vi "Get Channels Timing.vi"(8 "error in (no error)":errorcluster, 10 "group name in":string, 11 "Data file":T2) -> (0 "error out":errorcluster, 2 "Channels info":T1[](array[typedef]), 4 "Latest finish":dbl, 5 "Plots exist":bool, 6 "Earliest start":dbl)   [LabVIEW 2015]
uses:
  Controls/Channel name entry.ctl
  Controls/Data Viewer Entry.ctl
  Controls/TDMS channel info.ctl
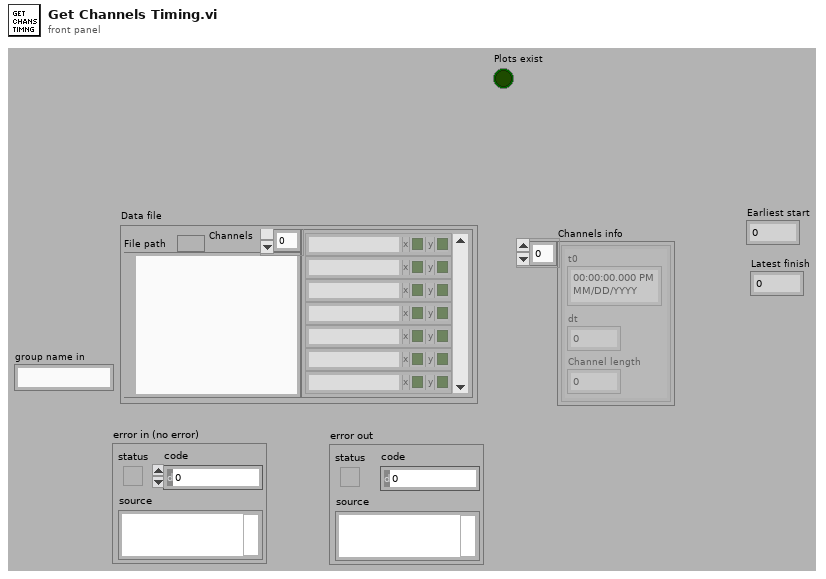
[diagram p1: front panel]
types:
  T1 = typedef "TDMS channel info.ctl" = cluster{"t0":timestamp, "dt":dbl, "Channel length":i64}
  T2 = typedef "Data Viewer Entry.ctl" = cluster{"File path":path, "Channels":T3[]}
  T3 = typedef "Channel name entry.ctl" = cluster{"Name":string, "x":bool, "y":bool}
  T4 = enum16{"open", "open or create", "create or replace", "create", "open (read-only)"}
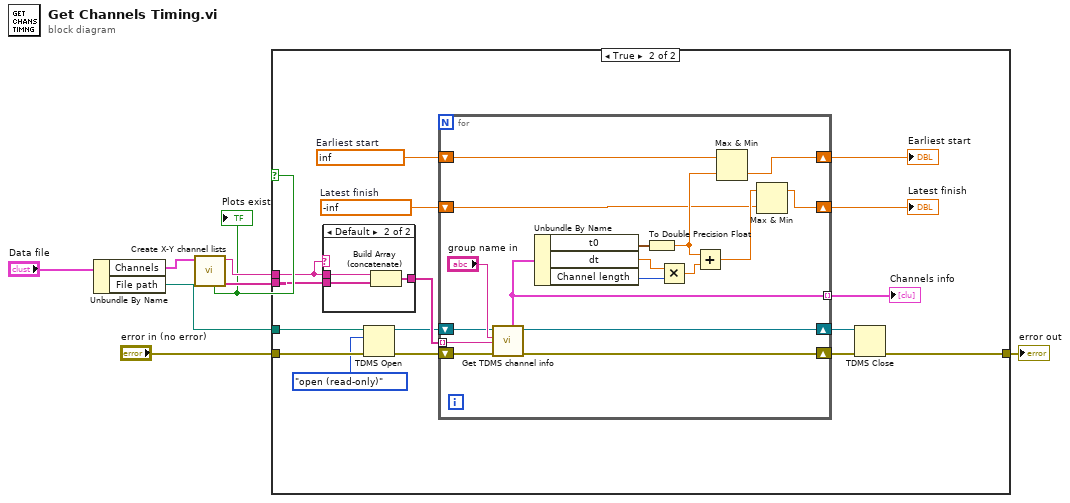
[diagram p0: block diagram]
diagram:
  n1 = Unbundle By Name("Data file") -> ("Channels"=w6:T3[], "File path"=w7:path)
  n2 = call "Create X-Y channel lists.vi"("Channels to plot"=w6) -> ("Y names"=w4:string[], "X-axis name"=w5:string, "Plots exist"=w1:bool)  [unwired: 6 in, 2 out]
  "Plots exist" <- w1
  n3 = case shown="True" w1 {
    tunnel: w7 -> [_ w25]
    tunnel: w5 -> [_ w11]
    tunnel: w4 -> [_ w23]
    tunnel: "error in (no error)" -> [w9 w13]
    tunnel: [w9 w12] -> w2
    frame False {
    }
    frame True {
      w18 = -inf  # Latest finish
      w19 = inf  # Earliest start
      n4 = case shown="Default" w11 {
        tunnel: w11 -> [_ w29]
        tunnel: w23 -> [w26 w28]
        tunnel: [w26 w27] -> w22
        frame "Time" {
        }
        frame Default {
          n5 = Build Array (concatenate)(w29, w28) -> (w27:string[])
        }
      }
      n6 = TDMS Open(8:w13, 10:T4."open (read-only)" ("operation (0:open)"), 11:w25) -> (0:w24:errorcluster, 3:w21:refnum<k34>)  [unwired: 4 in]
      n7 = for {
        tunnel: w22 -> [w44] mode=indexing
        shift-right: [w42] -> w15
        shift-left: w24 -> [w46]
        tunnel: [w40] -> w20 mode=indexing
        shift-right: [w37] -> w17
        shift-left: w19 -> [w38]
        shift-right: [w30] -> w16
        shift-left: w18 -> [w31]
        shift-right: [w41] -> w14
        shift-left: w21 -> [w43]
        n8 = call "Get TDMS channel info.vi"("error in"=w46, "Channel name"=w44, "group name"="group name in", "tdms file"=w43) -> ("error out"=w42:errorcluster, "tdms file out"=w41:refnum<k34>, "TDMS channel info"=w40:T1)  [unwired: 3 in, 2 out]
        n9 = Unbundle By Name(w40) -> ("t0"=w39:timestamp, "dt"=w36:dbl, "Channel length"=w35:i64)
        n10 = To Double Precision Float(number=w39) -> (double precision float=w34:dbl)
        n11 = Multiply(x=w36, y=w35) -> (x*y=w33:dbl)
        n12 = Add(x=w34, y=w33) -> (x+y=w32:dbl)
        n13 = Max & Min(x=w38, y=w34) -> (min(x,y)=w37:dbl)  [unwired: 1 out]
        n14 = Max & Min(x=w32, y=w31) -> (max(x,y)=w30:dbl)  [unwired: 1 out]
      }
      "Channels info" <- w20
      "Earliest start" <- w17
      "Latest finish" <- w16
      n15 = TDMS Close(8:w15, 11:w14) -> (0:w12:errorcluster)  [unwired: 1 out]
    }
  }
  "error out" <- w2
